vi "Update Data Plot.vi"(6 "Sample Rate (sec/sample)":dbl, 8 "Time interval (s)":i32, 9 "Instrument State":T2={"Data Directory"=path "", "Last Report Number"=0, "Yield"=0.0, "Max Concentration (mM)"=1.0, "Report File Pattern"="", "Current Data File"=path "", "Peak Data Array"=[], "Average Peak Data"={"Time Stamp"=timestamp(0 s since 1904-01-01), "Peaks"=[]}, "Points to Average"=3}, 11 "Graph History Arrays in":T1) -> (0 "Updated Graph History":cluster{timestamp[], dbl[]}[](array[cluster]), 3 "Graph History Arrays out":T1)   [LabVIEW 2020, in "Mock LC Parser.lvlib"]
uses:
  Mock LC Parser.lvlib
  Instrument Manager/Instrument State.ctl
  Instrument Manager/Instrument Manager.lvlib
  support/Data Display Loop Data.ctl
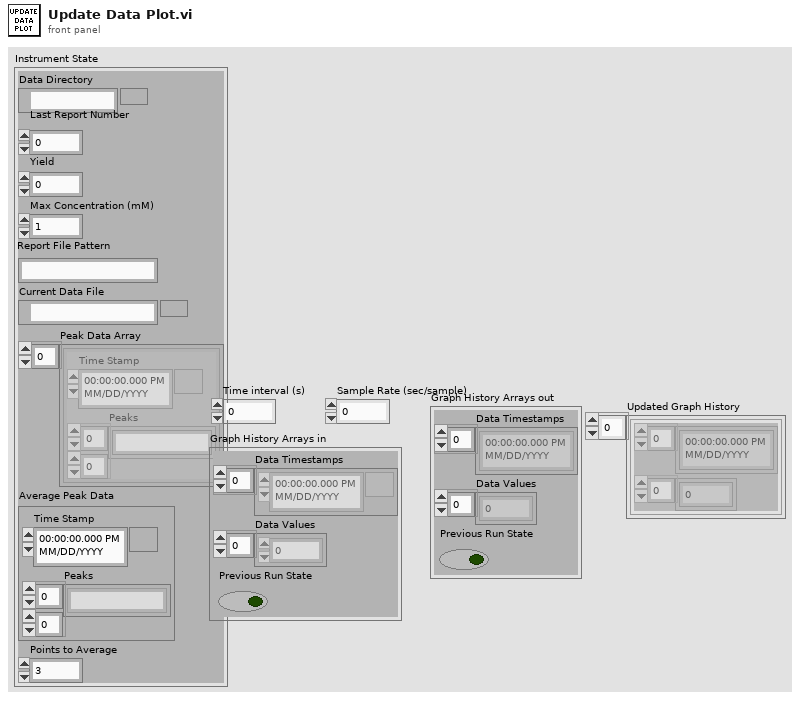
[diagram p1: front panel]
types:
  T1 = typedef "Mock LC Parser.lvlib/Data Display Loop Data.ctl" = cluster{"Data Timestamps":timestamp[], "Data Values":dbl[], "Previous Run State":bool}
  T2 = typedef "Mock LC Parser.lvlib/Instrument Manager.lvlib/Instrument State.ctl" = cluster{"Data Directory":path, "Last Report Number":i32, "Yield":dbl, "Max Concentration (mM)":dbl, "Report File Pattern":string, "Current Data File":path, "Peak Data Array":cluster{"Time Stamp":timestamp, "Peaks":string[][]}[], "Average Peak Data":cluster{"Time Stamp":timestamp, "Peaks":string[][]}, "Points to Average":i32}
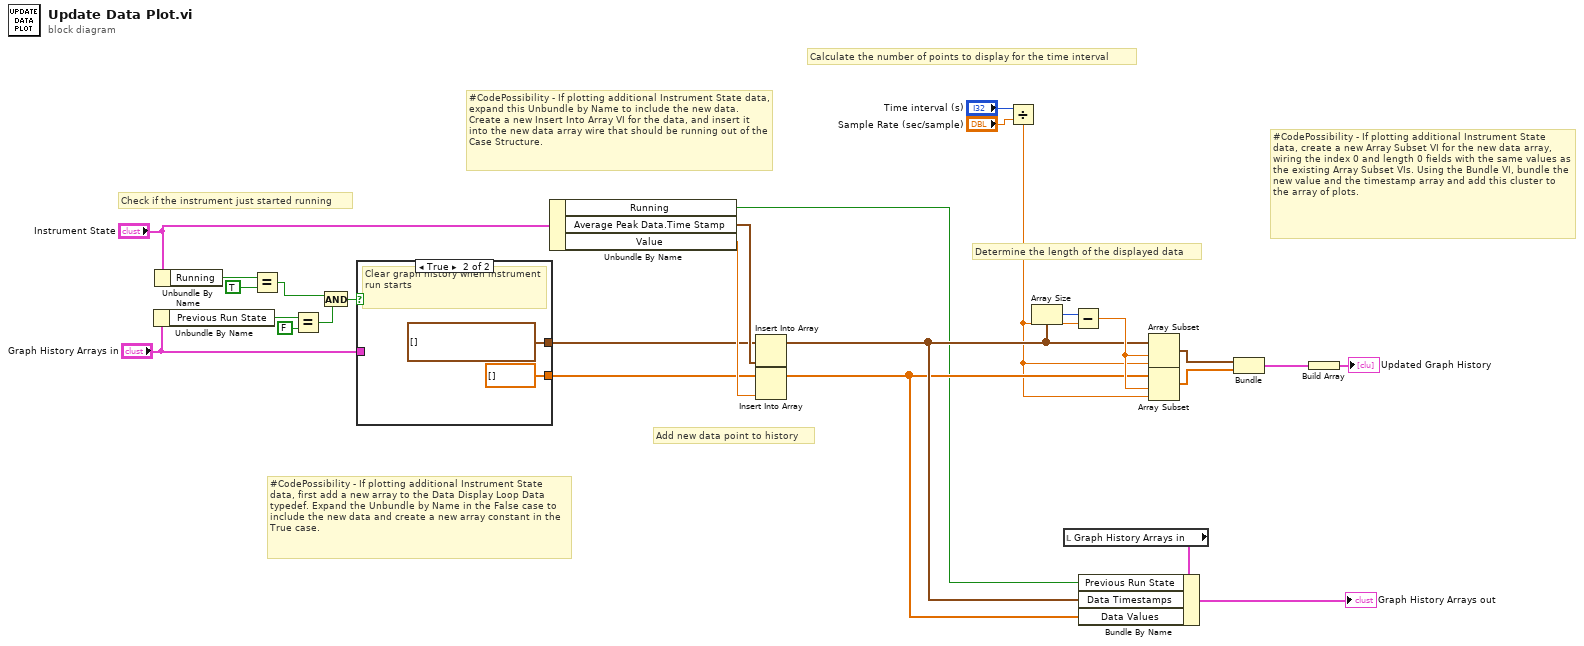
[diagram p0: block diagram]
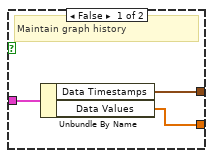
[diagram p2: hidden frame]
diagram:
  # "#CodePossibility - If plotting additional Instrument State data, create a new Array Subset VI for the new data array, wiring the index 0 and length 0 fields with the same values as the existing Array Subset VIs. Using the Bundle VI, bundle the new value and the timestamp array and add this cluster to the array of plots."
  # "#CodePossibility - If plotting additional Instrument State data, expand this Unbundle by Name to include the new data. Create a new Insert Into Array VI for the data, and insert it into the new data array wire that should be running out of the Case Structure."
  # "#CodePossibility - If plotting additional Instrument State data, first add a new array to the Data Display Loop Data typedef. Expand the Unbundle by Name in the False case to include the new data and create a new array constant in the True case."
  # "Check if the instrument just started running"
  # "Add new data point to history"
  # "Calculate the number of points to display for the time interval"
  # "Determine the length of the displayed data"
  n1 = Unbundle By Name("Graph History Arrays in") -> ("Previous Run State"=w8:bool)
  n2 = Unbundle By Name("Instrument State") -> ("Running"=w18:bool)
  n3 = Equal?(x=w18, y=TRUE) -> (x = y?=w4:bool)
  n4 = Equal?(x=w8, y=FALSE) -> (x = y?=w5:bool)
  n5 = And(x=w4, y=w5) -> (x .and. y?=w6:bool)
  n6 = case shown="True" w6 {
    tunnel: "Graph History Arrays in" -> [w30 _]
    tunnel: [w29 dbl[] [] ("Data Values")] -> w11
    tunnel: [w28 timestamp[] [] ("Data Timestamps")] -> w10
    frame False {
      # "Maintain graph history"
      n7 = Unbundle By Name(w30) -> ("Data Timestamps"=w28:timestamp[], "Data Values"=w29:dbl[])
    }
    frame True {
      # "Clear graph history when instrument run starts"
    }
  }
  n8 = Unbundle By Name("Instrument State") -> ("Running"=w3:bool, "Average Peak Data.Time Stamp"=w13:timestamp, "Value"=w12:dbl)
  n9 = Insert Into Array(array=w10, new element=w13) -> (w17:timestamp[])  [unwired: 1 in]
  n10 = Insert Into Array(array=w11, new element=w12) -> (w16:dbl[])  [unwired: 1 in]
  n11 = Divide(x="Time interval (s)", y="Sample Rate (sec/sample)") -> (x/y=w15:dbl)
  n12 = Array Size(array=w17) -> (size(s)=w25:i32)
  n13 = local read "Graph History Arrays in"() -> (w14:T1)
  n14 = Subtract(x=w25, y=w15) -> (x-y=w24:dbl)
  n15 = Bundle By Name(cluster=w14, "Previous Run State"=w3, "Data Timestamps"=w17, "Data Values"=w16) -> (→"Graph History Arrays out":T1)
  n16 = Array Subset(array=w17, index=w24, length=w15) -> (w23:timestamp[])
  n17 = Array Subset(array=w16, index=w24, length=w15) -> (w22:dbl[])
  n18 = Bundle(w23, w22) -> (w2:cluster{timestamp[], dbl[]})  [unwired: 1 in]
  n19 = Build Array(w2) -> (→"Updated Graph History":cluster{timestamp[], dbl[]}[])
